vi "LaserInitialize.vi"() -> (3 "client handle out":T1)   [LabVIEW 2020]
uses:
  <vilib>/httpClient/ClientHandle.ctl
  <vilib>/httpClient/LabVIEWHTTPClient.lvlib
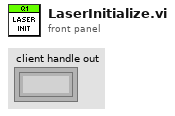
[diagram p1: front panel]
types:
  T1 = typedef "LabVIEWHTTPClient.lvlib/ClientHandle.ctl" = refnum<k1>
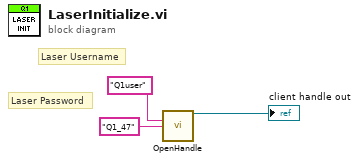
[diagram p0: block diagram]
diagram:
  # "Laser Password"
  # "Laser Username"
  n1 = call <vilib>:"OpenHandle.vi"("username"="Q1user", "password"="Q1_47") -> ("client handle out"=→"client handle out":T1)  [unwired: 12 in, 1 out]
